vi "Call Popup Message.vi"(1 "error in":errorcluster, 2 "Button Text":string, 3 "Dialogue Message":string) -> (0 "error out":errorcluster)   [LabVIEW 2025]
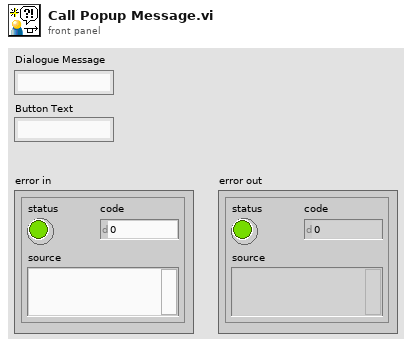
[diagram p1: front panel]
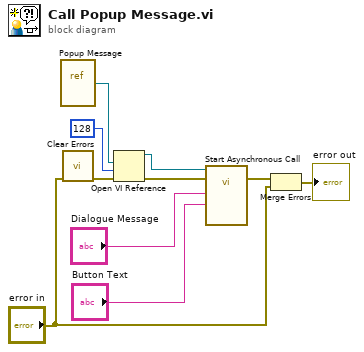
[diagram p0: block diagram]
diagram:
  n1 = vi-ref "Popup Message.vi"() -> (w5:refnum<vi>)
  n2 = call <vilib>:"Clear Errors.vi"("error in (no error)"="error in") -> ("error out"=w2:errorcluster)  [unwired: 5 in, 1 out]
  n3 = Open VI Reference(vi path=w5, options=128, error in (no error)=w2) -> (vi reference=w4:refnum<vi>, error out=w1:errorcluster)  [unwired: 3 in]
  n4 = call-by-ref "Start Asynchronous Call"(reference=w4, error in=w1, "Button Name"="Button Text", "Dialogue Message"="Dialogue Message") -> (error out=w10:errorcluster)  [unwired: 1 in, 2 out]
  n5 = Merge Errors(w10, "error in") -> (→"error out":errorcluster)
